vi "GetSourceData.vi"(8 "error in (no error)":errorcluster, 11 "ChildSource in":refnum<class "ChildSource.lvclass">) -> (0 "error out":errorcluster, 2 "SourceData":dbl, 3 "ChildSource out":refnum<class "ChildSource.lvclass">)   [LabVIEW 2023, in "ChildSource.lvclass"]
uses:
  ChildSource.lvclass
  ChildSource.lvclass/ChildSource.ctl
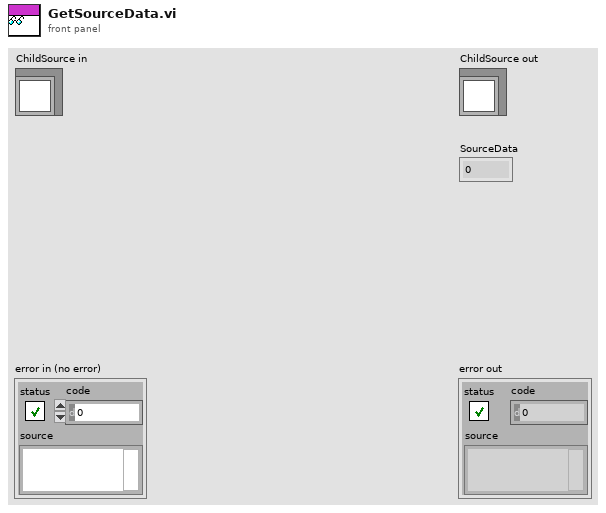
[diagram p1: front panel]
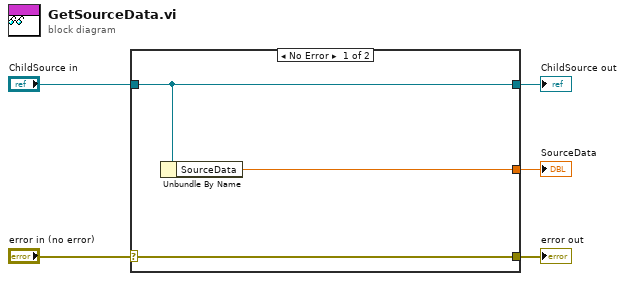
[diagram p0: block diagram]
diagram:
  n1 = case shown="No Error" "error in (no error)" {
    selector: "error in (no error)" -> [w8 w9]
    tunnel: [w8 w9] -> w4
    tunnel: [w7 w10] -> w2
    tunnel: "ChildSource in" -> [w7 w10]
    tunnel: [w6 _] -> w1
    frame No Error {
      n2 = Unbundle By Name(w7) -> ("SourceData"=w6:dbl)
    }
    frame Error {
    }
  }
  "error out" <- w4
  "ChildSource out" <- w2
  "SourceData" <- w1
